vi "NI VeriStand - Receive Packet from Host.vi"(11 "Prev":bool) -> (0 "Next":bool, 1 "Element":u64)   [LabVIEW 2020, in "NI_VS FPGA Support.lvlib"]
uses:
  <vilib>/NI VeriStand/FPGA/NI_VS FPGA Support.lvlib
  <vilib>/rvi/DataTransferAndStorage/Container/XNode/niFpgaContainer.xnode
  <vilib>/rvi/interface/RandomDataEmulation/nirviRandomDataFpgaReadWriteTemplate.vi
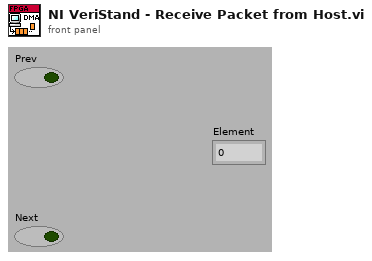
[diagram p1: front panel]
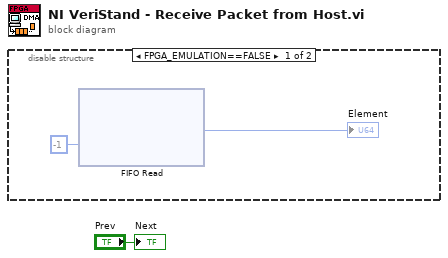
[diagram p0: block diagram]
diagram:
  n1 = disable-structure shown="FPGA_EMULATION==FALSE" {
    frame condition #0 {
      n2 = xnode ("FIFO Read")("Timeout"=-1) -> ("Element"=→"Element":u64)  [unwired: 1 in, 2 out]
    }
    frame condition #1 (active) {
    }
  }
  "Next" <- "Prev"
